vi "UIRef.vi"(8 "error in":errorcluster, 11 "node in":refnum<class "CI Project.lvclass">) -> (0 "error out":errorcluster, 2 "VI refnum":refnum<vi>, 3 "node out":refnum<class "CI Project.lvclass">)   [LabVIEW 2014, in "CI Project.lvclass"]
doc: "Stores the static reference to the UI of the node."
uses:
  CI Project.lvclass
  CI Project UI.vi
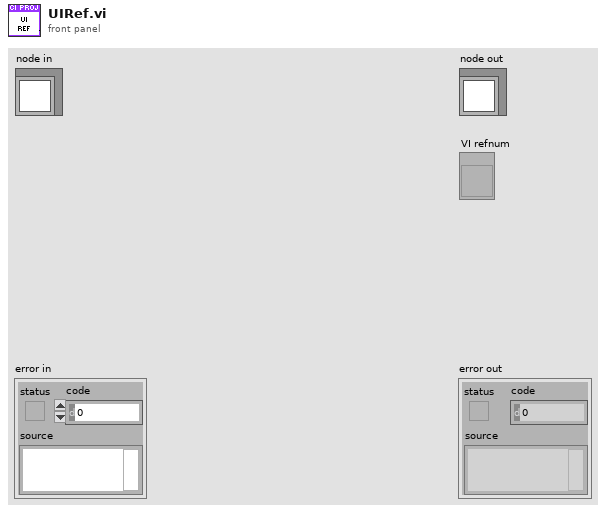
[diagram p1: front panel]
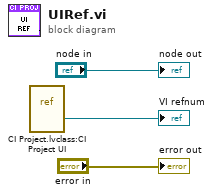
[diagram p0: block diagram]
diagram:
  n1 = vi-ref "CI Project.lvclass:CI Project UI.vi"() -> (→"VI refnum":refnum<vi>)
  "error out" <- "error in"
  "node out" <- "node in"
